vi "TestImport.vi"() -> ()   [LabVIEW 2021]
uses:
  ErrorDefinitionSQLite/ErrorContent.ctl
  ErrorDefinitionSQLite/ErrorDefinitionSQLite.lvclass
panel:
  in  "ErrorsNotInDatabase":T1
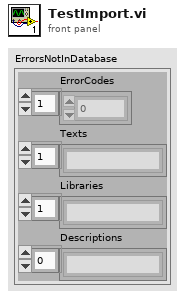
[diagram p1: front panel]
types:
  T1 = typedef "ErrorDefinitionSQLite.lvclass/ErrorContent.ctl" = cluster{"ErrorCodes":i32[], "Texts":string[], "Libraries":string[], "Descriptions":string[]}
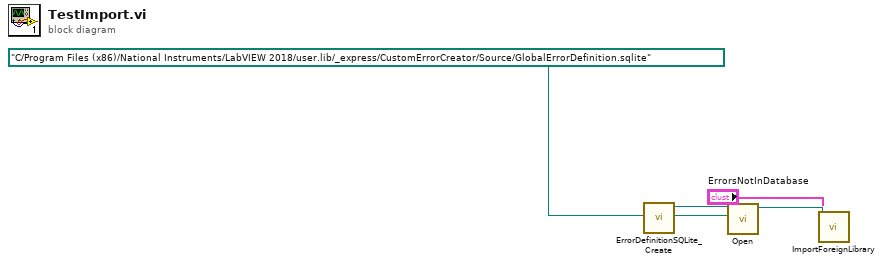
[diagram p0: block diagram]
diagram:
  n1 = call "ErrorDefinitionSQLite_Create.vi"() -> ("Reference out"=w4:refnum<class "ErrorDefinitionSQLite.lvclass">)  [unwired: 10 in, 1 out]
  n2 = call-dynamic "Open.vi"("Path"=path "C:/Program Files (x86)/National Instruments/LabVIEW 2018/user.lib/_express/CustomErrorCreator/Source/GlobalErrorDefinition.sqlite", "ReferenceIn"=w4) -> ("ReferenceOut"=w2:refnum<class "ErrorDefinitionSQLite.lvclass">)  [unwired: 8 in, 1 out]
  n3 = call "ImportForeignLibrary.vi"("ErrorsNotInDatabase"="ErrorsNotInDatabase", "ReferenceIn"=w2) -> ()  [unwired: 9 in, 1 out]
